vi "CheckPauseBetweenTimeString.vi"(8 "greater than (s)":dbl=60.0, 10 "laterEntry":string[](array[string])=["15:54", "902_3218_call1", "3", "2,5", "3"], 11 "earlierEntry":string[](array[string])=["15:53", "902_3218_call1", "3", "2,5", "3"]) -> (0 "pause ok":bool, 3 "pause":dbl=60.0)   [LabVIEW 2014]
panel:
  out "output 2":timestamp=timestamp(53580 s since 1904-01-01)
  out "output 1":timestamp=timestamp(53640 s since 1904-01-01)
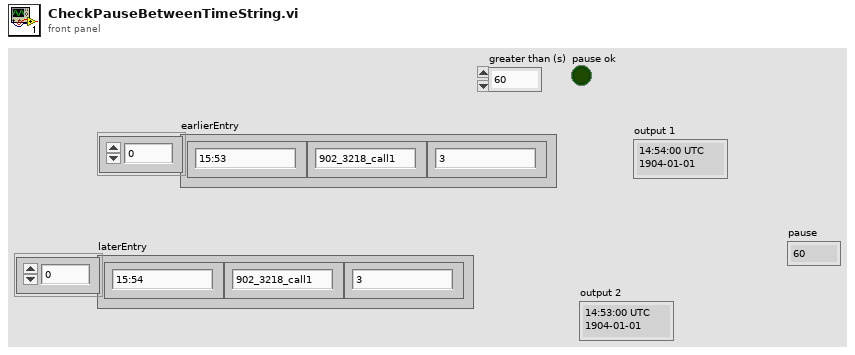
[diagram p1: front panel]
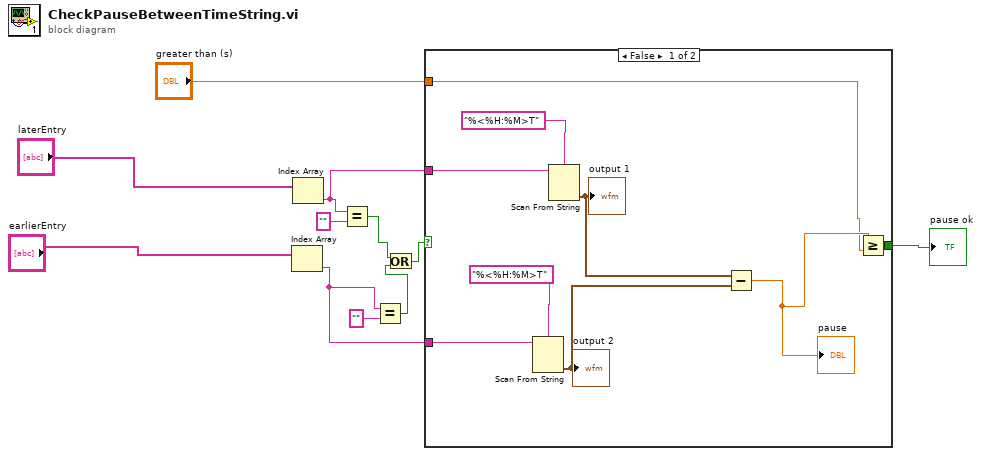
[diagram p0: block diagram]
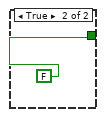
[diagram p2: hidden frame]
diagram:
  n1 = Index Array(array="earlierEntry") -> (element=w4:string)  [unwired: 1 in]
  n2 = Index Array(array="laterEntry") -> (element=w7:string)  [unwired: 1 in]
  n3 = Equal?(x=w7, y="") -> (x = y?=w3:bool)
  n4 = Equal?(x=w4, y="") -> (x = y?=w1:bool)
  n5 = Or(x=w3, y=w1) -> (x .or. y?=w2:bool)
  n6 = case shown="False" w2 {
    tunnel: w7 -> [w19 _]
    tunnel: w4 -> [w17 _]
    tunnel: "greater than (s)" -> [w12 _]
    tunnel: [w14 FALSE] -> w8
    frame False {
      n7 = Scan From String(format string="%<%H:%M>T", input string=w17) -> (output 1=w15:timestamp)  [unwired: 3 in, 3 out]
      "output 2" <- w15
      n8 = Scan From String(format string="%<%H:%M>T", input string=w19) -> (output 1=w16:timestamp)  [unwired: 3 in, 3 out]
      "output 1" <- w16
      n9 = Subtract(x=w16, y=w15) -> (x-y=w13:dbl)
      "pause" <- w13
      n10 = Greater Or Equal?(x=w13, y=w12) -> (x >= y?=w14:bool)
    }
    frame True {
    }
  }
  "pause ok" <- w8
